vi "URG-04LX-UG01 Read Measurement Data.vi"(8 "error in":errorcluster, 9 "Acquisition Parameters":T1, 11 "VISA Refnum in":refnum<visa-resource-name>) -> (0 "error out":errorcluster, 1 "Acquisition Parameters":T1, 2 "Distance Measurements":i32[](array[numeric]), 3 "VISA Refnum out":refnum<visa-resource-name>)   [LabVIEW 2018]
doc: "Processes any returned data from a connected Hokuyo URG-04LX-UG01 device and returns an array of distance measurements in millimeters via the <b>Distance Measurements</b> indicator."
uses:
  Type Definitions/Acquisition Parameters.ctl
  Type Definitions/Measurement Type.ctl
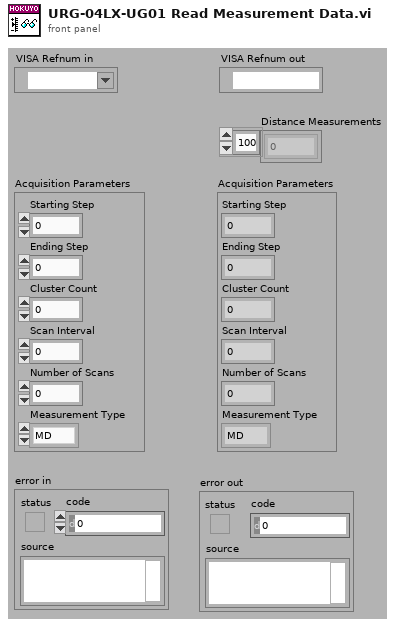
[diagram p1: front panel]
types:
  T1 = typedef "Acquisition Parameters.ctl" = cluster{"Starting Step":i32, "Ending Step":i32, "Cluster Count":i32, "Scan Interval":i32, "Number of Scans":i32, "Measurement Type":T2}
  T2 = typedef "Measurement Type.ctl" = enum16{"MD", "MS"}
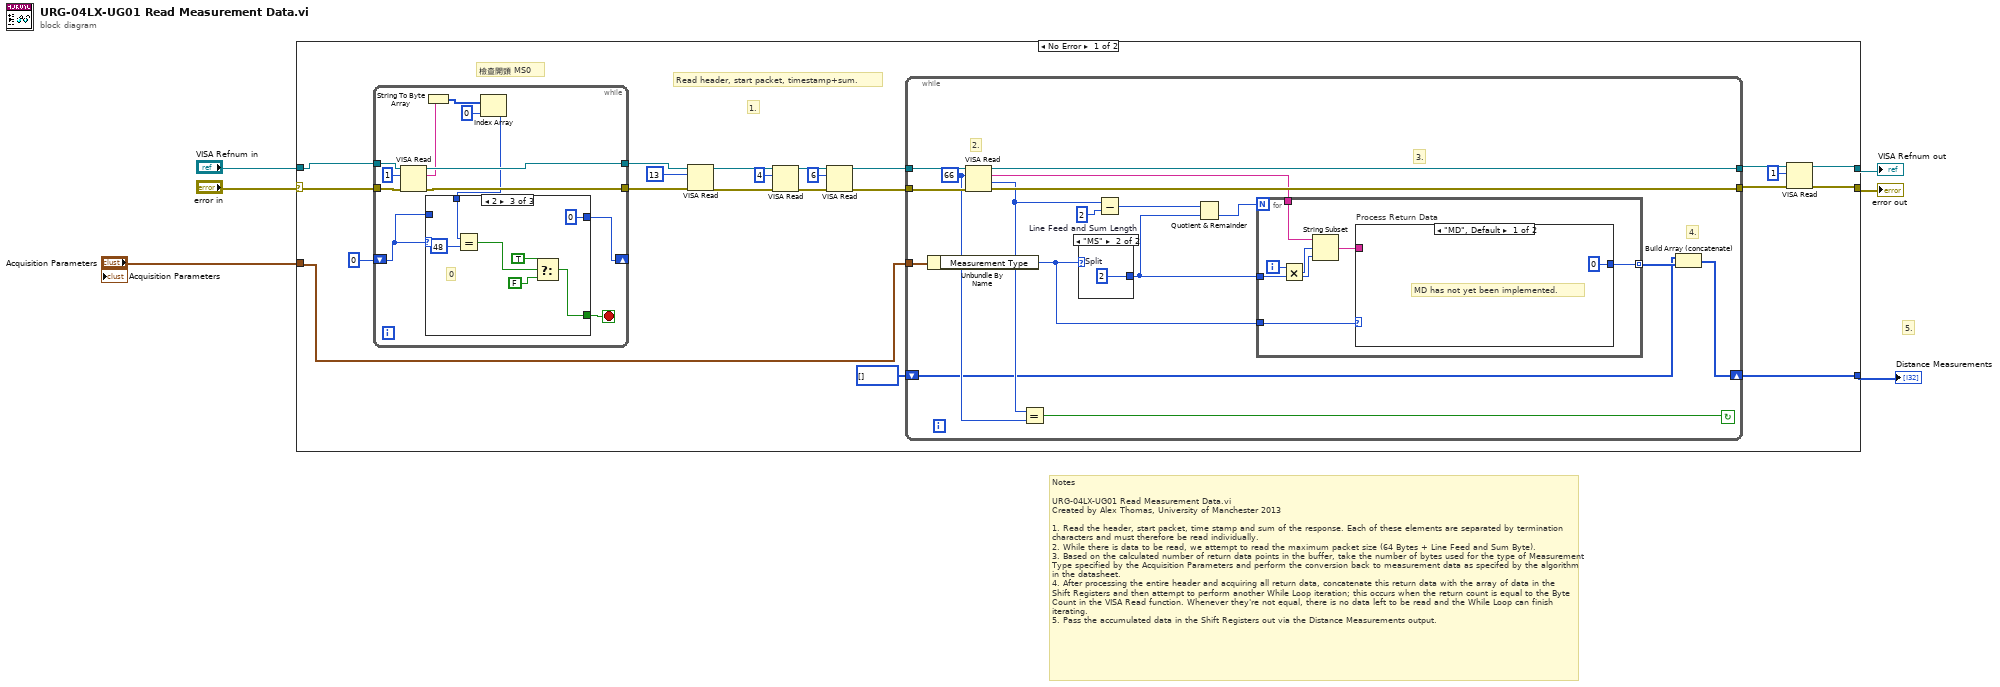
[diagram p0: block diagram]
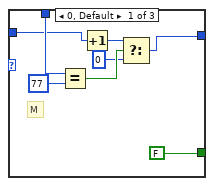
[diagram p2: hidden frame]
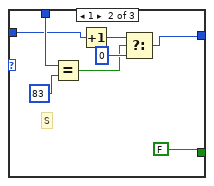
[diagram p3: hidden frame]
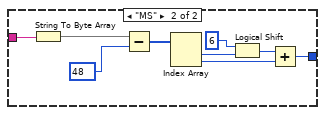
[diagram p4: hidden frame]
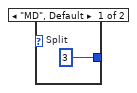
[diagram p5: hidden frame]
diagram:
  # "Notes\n\nURG-04LX-UG01 Read Measurement Data.vi\nCreated by Alex Thomas, University of Manchester 2013\n\n1. Read the header, start packet, time stamp and sum of the response. Each of these elements are separated by termination characters and must therefore be read individually. \n2. While there is data to be read, we attempt to read the maximum packet size (64 Bytes + Line Feed and Sum Byte).\n3. Based on the calculated number of return data points in the buffer, take the number of bytes used for the type of Measurement Type specified by the Acquisition Parameters and perform the conversion back to measurement data as specifed by the algorithm in the datasheet.\n4. After processing the entire header and acquiring all return data, concatenate this return data with the array of data in the Shift Registers and then attempt to perform another While Loop iteration; this occurs when the return count is equal to the Byte Count in the VISA Read function. Whenever they're not equal, there is no data left to be read and the While Loop can finish iterating.\n5. Pass the accumulated data in the Shift Registers out via the Distance Measurements output."
  # "5."
  n1 = case shown="No Error" "error in" {
    selector: "error in" -> [w11 w101]
    tunnel: "Acquisition Parameters" -> [w8 _]
    tunnel: [w15 w101] -> w6
    tunnel: [w14 w100] -> w5
    tunnel: "VISA Refnum in" -> [w12 w100]
    tunnel: [w18 _] -> w2
    frame No Error {
      # "檢查開頭 MS0"
      # "1."
      # "Read header, start packet, timestamp+sum."
      n2 = while {
        tunnel: w12 -> [w40]
        tunnel: [w38] -> w10
        tunnel: w11 -> [w39]
        tunnel: [w37] -> w9
        shift-right: [w35] -> _
        shift-left: 0 -> [w34]
        stop <- w29 stop-if-true
        n3 = VISA Read(VISA resource name=w40, byte count=u32 1, error in (no error)=w39) -> (VISA resource name out=w38:refnum<visa-resource-name>, read buffer=w33:string, error out=w37:errorcluster)  [unwired: 1 out]
        n4 = String To Byte Array(string=w33) -> (unsigned byte array=w32:u8[])
        n5 = Index Array(array=w32, index=0) -> (element=w30:u8)
        n6 = case shown="2" w34 {
          tunnel: [w45 w52 0 ("f")] -> w35
          tunnel: w34 -> [w44 w54 _]
          tunnel: w30 -> [w48 w56 w63]
          tunnel: [FALSE FALSE w58] -> w29
          frame 0, Default {
            # "M"
            n7 = Equal?(x=w48, y=u8 77) -> (x = y?=w43:bool)
            n8 = Increment(x=w44) -> (x+1=w46:i32)
            n9 = Select(t=w46, s=w43, f=0) -> (s? t:f=w45:i32)
          }
          frame 1 {
            # "S"
            n10 = Equal?(x=w56, y=u8 83) -> (x = y?=w50:bool)
            n11 = Increment(x=w54) -> (x+1=w53:i32)
            n12 = Select(t=w53, s=w50, f=0) -> (s? t:f=w52:i32)
          }
          frame 2 {
            # "0"
            n13 = Equal?(x=w63, y=u8 48) -> (x = y?=w61:bool)
            n14 = Select(t=TRUE, s=w61, f=FALSE) -> (s? t:f=w58:bool)
          }
        }
      }
      n15 = VISA Read(VISA resource name=w10, byte count=u32 13, error in (no error)=w9) -> (VISA resource name out=w21:refnum<visa-resource-name>, error out=w22:errorcluster)  [unwired: 2 out]
      n16 = VISA Read(VISA resource name=w21, byte count=u32 4, error in (no error)=w22) -> (VISA resource name out=w24:refnum<visa-resource-name>, error out=w25:errorcluster)  [unwired: 2 out]
      n17 = VISA Read(VISA resource name=w24, byte count=u32 6, error in (no error)=w25) -> (VISA resource name out=w26:refnum<visa-resource-name>, error out=w27:errorcluster)  [unwired: 2 out]
      n18 = while {
        tunnel: w26 -> [w80]
        tunnel: w27 -> [w79]
        tunnel: [w78] -> w17
        tunnel: [w77] -> w16
        tunnel: w8 -> [w74]
        shift-right: [w65] -> w18
        shift-left: i32[] [] -> [w64]
        stop <- w75 continue-if-true
        w69 = u32 2  # Line Feed and Sum Length
        w76 = u32 66 ("byte count")
        # "4."
        # "3."
        # "2."
        n19 = Unbundle By Name(w74) -> ("Measurement Type"=w67:T2)
        n20 = VISA Read(VISA resource name=w80, byte count=w76, error in (no error)=w79) -> (VISA resource name out=w78:refnum<visa-resource-name>, read buffer=w72:string, return count=w73:u32, error out=w77:errorcluster)
        n21 = Equal?(x=w73, y=w76) -> (x = y?=w75:bool)
        n22 = case shown="\"MS\"" w67 {
          tunnel: [w98 w99] -> w71
          frame "MD", Default {
            w98 = u32 3  # Split
          }
          frame "MS" {
            w99 = u32 2  # Split
          }
        }
        n23 = Subtract(x=w73, y=w69) -> (x-y=w70:u32)
        n24 = Quotient & Remainder(x=w70, y=w71) -> (floor(x/y)=w68:u32)  [unwired: 1 out]
        n25 = for {
          N: w68 -> [_]
          tunnel: w72 -> [w87]
          tunnel: w71 -> [w84]
          tunnel: w67 -> [w83]
          tunnel: [w81] -> w66 mode=indexing
          i -> [w85]
          n26 = Multiply(x=w85, y=w84) -> (x*y=w86:u32)
          n27 = String Subset(string=w87, offset (0)=w86, length (rest)=w84) -> (substring=w82:string)
          n28 = case "Process Return Data" shown="\"MD\", Default" w83 {
            tunnel: w82 -> [_ w97]
            tunnel: [0 w89] -> w81
            frame "MD", Default {
              # "MD has not yet been implemented."
            }
            frame "MS" {
              n29 = String To Byte Array(string=w97) -> (unsigned byte array=w96:u8[])
              n30 = Subtract(x=w96, y=48) -> (x-y=w94:i32[])
              n31 = Index Array(array=w94) -> (element #1=w93:i32, element #2=w90:i32)  [unwired: 2 in]
              n32 = Logical Shift(y=i8 6, x=w93) -> (x << y=w91:i32)
              n33 = Add(x=w91, y=w90) -> (x+y=w89:i32)
            }
          }
        }
        n34 = Build Array (concatenate)(w64, w66) -> (w65:i32[])
      }
      n35 = VISA Read(VISA resource name=w17, byte count=u32 1, error in (no error)=w16) -> (VISA resource name out=w14:refnum<visa-resource-name>, error out=w15:errorcluster)  [unwired: 2 out]
    }
    frame Error {
    }
  }
  "error out" <- w6
  "VISA Refnum out" <- w5
  "Distance Measurements" <- w2
  "Acquisition Parameters" <- "Acquisition Parameters"
